vi "determineConfigurationDirectoryPathWindows.vi"(8 "error in (no error)":errorcluster, 11 "WindowsTarget in":refnum<class "cRIOScanModeTarget.lvclass">) -> (0 "error out":errorcluster, 2 "configDirectoryPathWindows":path, 3 "WindowsTarget out":refnum<class "cRIOScanModeTarget.lvclass">)   [LabVIEW 2012, in "cRIOScanModeTarget.lvclass"]
doc: "Returns the configuration directory path applicable on a Windows target based on the application directory. The implementation takes into account the application kind (Development System or Run-Time System)."
uses:
  cRIOScanModeTarget.lvclass
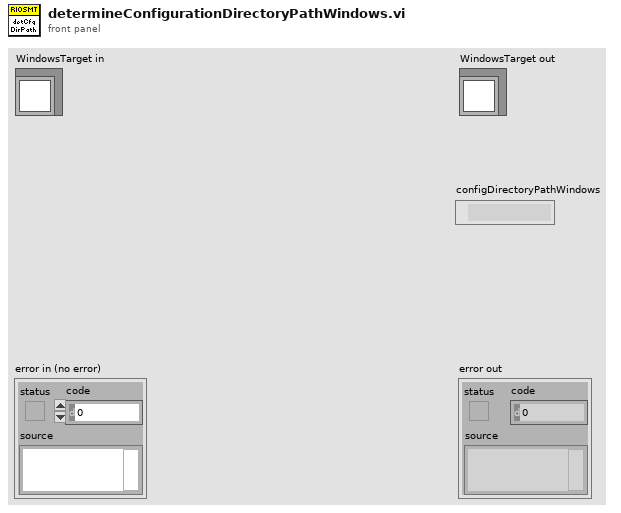
[diagram p1: front panel]
types:
  T1 = enum32{"invalid app kind", "Development System", "Run Time System", "Student Edition", "Embedded LabVIEW", "Evaluation", "Custom"}
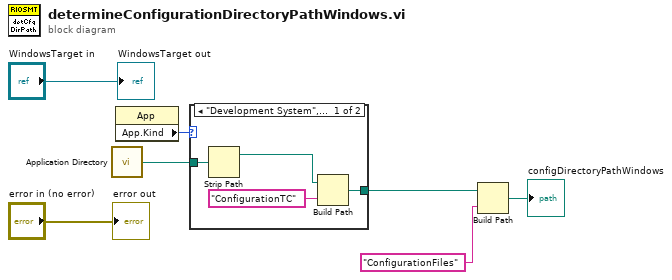
[diagram p0: block diagram]
diagram:
  n1 = call <vilib>:"Application Directory.vi"() -> ("Application Directory"=w3:path)
  n2 = property class="App"() -> ("App.Kind"=w2:T1)  [unwired: 2 in, 2 out]
  n3 = case shown="\"Development System\", Default" w2 {
    tunnel: [w10 w12] -> w5
    tunnel: w3 -> [w11 w12]
    frame "Development System", Default {
      n4 = Strip Path(path=w11) -> (stripped path=w9:path)  [unwired: 1 out]
      n5 = Build Path(base path=w9, name or relative path="ConfigurationTC") -> (appended path=w10:path)
    }
    frame "Run Time System" {
    }
  }
  n6 = Build Path(base path=w5, name or relative path="ConfigurationFiles") -> (appended path=→"configDirectoryPathWindows":path)
  "error out" <- "error in (no error)"
  "WindowsTarget out" <- "WindowsTarget in"
